vi "Wait for lifecycle state.vi"(8 "error in (no error)":errorcluster, 9 "Timeout [ms]":u32, 10 "Lifecycle State":T1, 11 "UI View in":refnum<class "View.lvclass">) -> (0 "error out":errorcluster, 3 "UI View out":refnum<class "View.lvclass">)   [LabVIEW 2020, in "View Dev Test.lvclass"]
uses:
  View Dev Test.lvclass
  source/Framework/Process/Public/Lifecycle/Lifecycle State.ctl
  source/Framework/View/View.lvclass
  C:/Git/astemes-triarc-framework/source/Framework/Process/Process.lvclass
  source/Framework/Process/Process.lvclass/Process.ctl
  <vilib>/Utility/error.llb/Clear Errors.vi
  source/Framework/Process/Process.lvclass
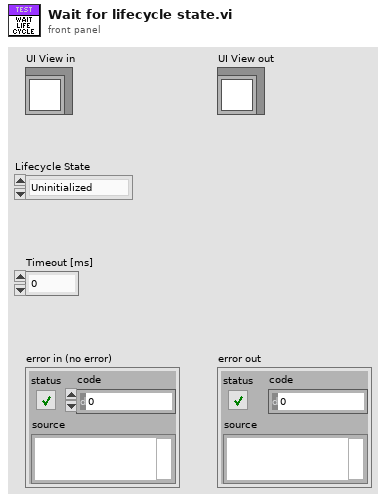
[diagram p1: front panel]
types:
  T1 = typedef "Process.lvclass/Lifecycle State.ctl" = enum16{"Uninitialized", "Initialized", "Started", "Running", "Stopped", "Finished"}
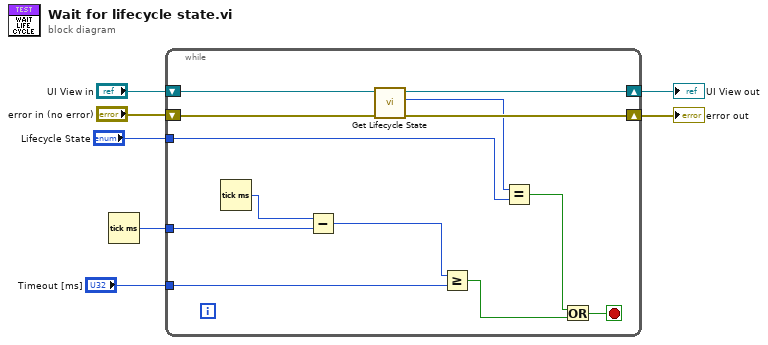
[diagram p0: block diagram]
diagram:
  n1 = Tick Count (ms)() -> (millisecond timer value=w2:u32)
  n2 = while {
    shift-right: [w19] -> w4
    shift-left: "UI View in" -> [w20]
    shift-right: [w17] -> w6
    shift-left: "error in (no error)" -> [w18]
    tunnel: "Lifecycle State" -> [w9]
    tunnel: w2 -> [w16]
    tunnel: "Timeout [ms]" -> [w13]
    stop <- w12 stop-if-true
    n3 = Tick Count (ms)() -> (millisecond timer value=w15:u32)
    n4 = Subtract(x=w15, y=w16) -> (x-y=w14:u32)
    n5 = call "Get Lifecycle State.vi"("error in (no error)"=w18, "Process In"=w20) -> ("error out"=w17:errorcluster, "Lifecycle State"=w10:T1, "Process Out"=w19:refnum<class "View.lvclass">)  [unwired: 6 in, 1 out]
    n6 = Greater Or Equal?(x=w14, y=w13) -> (x >= y?=w11:bool)
    n7 = Equal?(x=w10, y=w9) -> (x = y?=w8:bool)
    n8 = Or(x=w8, y=w11) -> (x .or. y?=w12:bool)
  }
  "error out" <- w6
  "UI View out" <- w4
